vi "flush_debug_fifo_all.vi"(8 "error in (no error)":errorcluster, 11 "Refnum in":T1) -> (0 "error out":errorcluster, 3 "Refnum out":T1)   [LabVIEW 2020]
uses:
  <vilib>/rvi/interface/nirviMethod/nirviMethod.xnode
  <vilib>/FPGAPlugInAG/Dynamic/niLvFpga_ReadFifo_Dynamic.vi
  <vilib>/rvi/errors/niLvFpgaMergeErrorWithErrorCode.vi
  RIG-SPECIFIC FILES/FPGA Refs/FPGA Ref.ctl
panel:
  out "Data 4":u32[](array[numeric])
  out "Elements Remaining 4":u32
  out "Elements Remaining 3":u32
  out "Data 3":u64[](array[numeric])
  out "Data 2":u8[](array[numeric])
  out "Elements Remaining 2":u32
  out "Data":u64[](array[numeric])
  out "Elements Remaining":u32
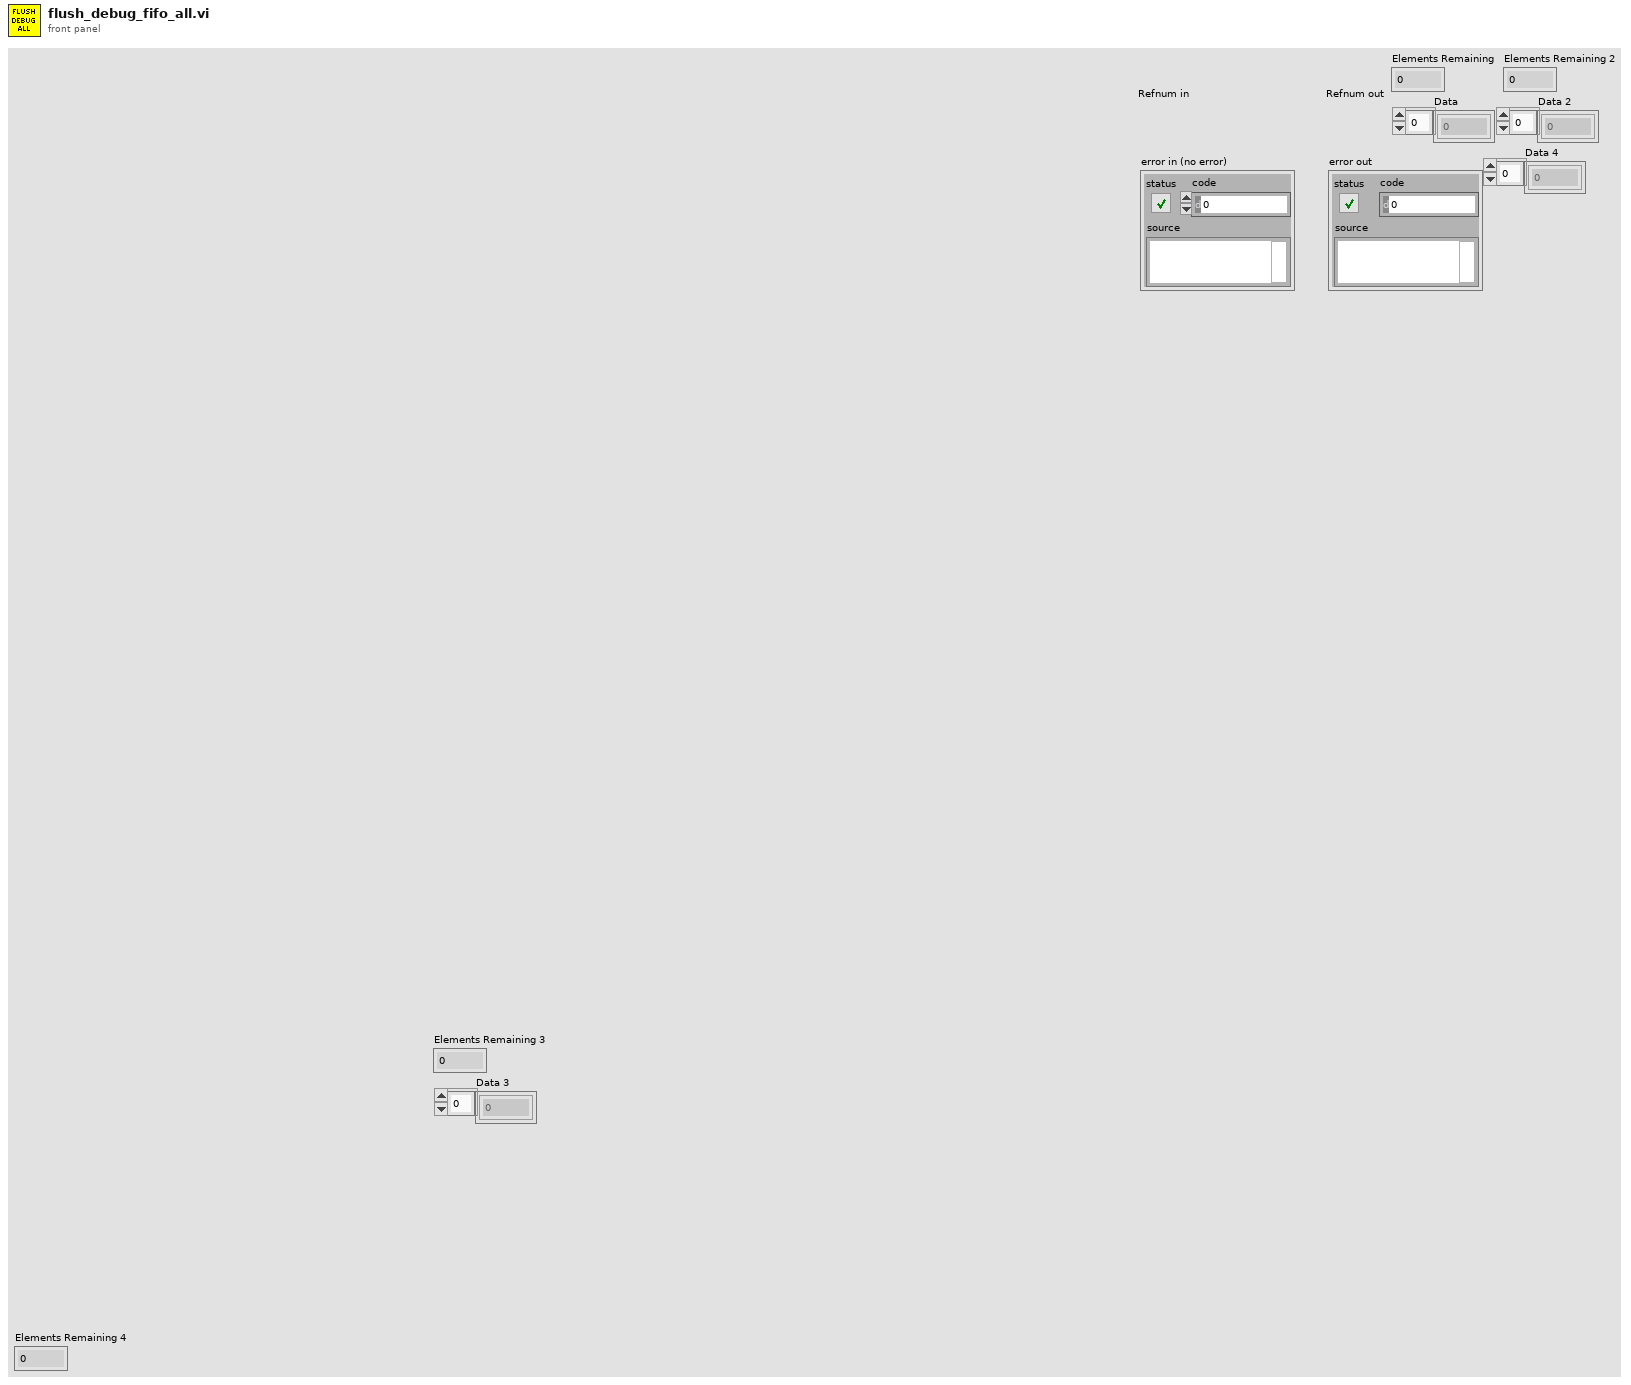
[diagram p1: front panel]
types:
  T1 = typedef "FPGA Ref.ctl" = refnum<k20>
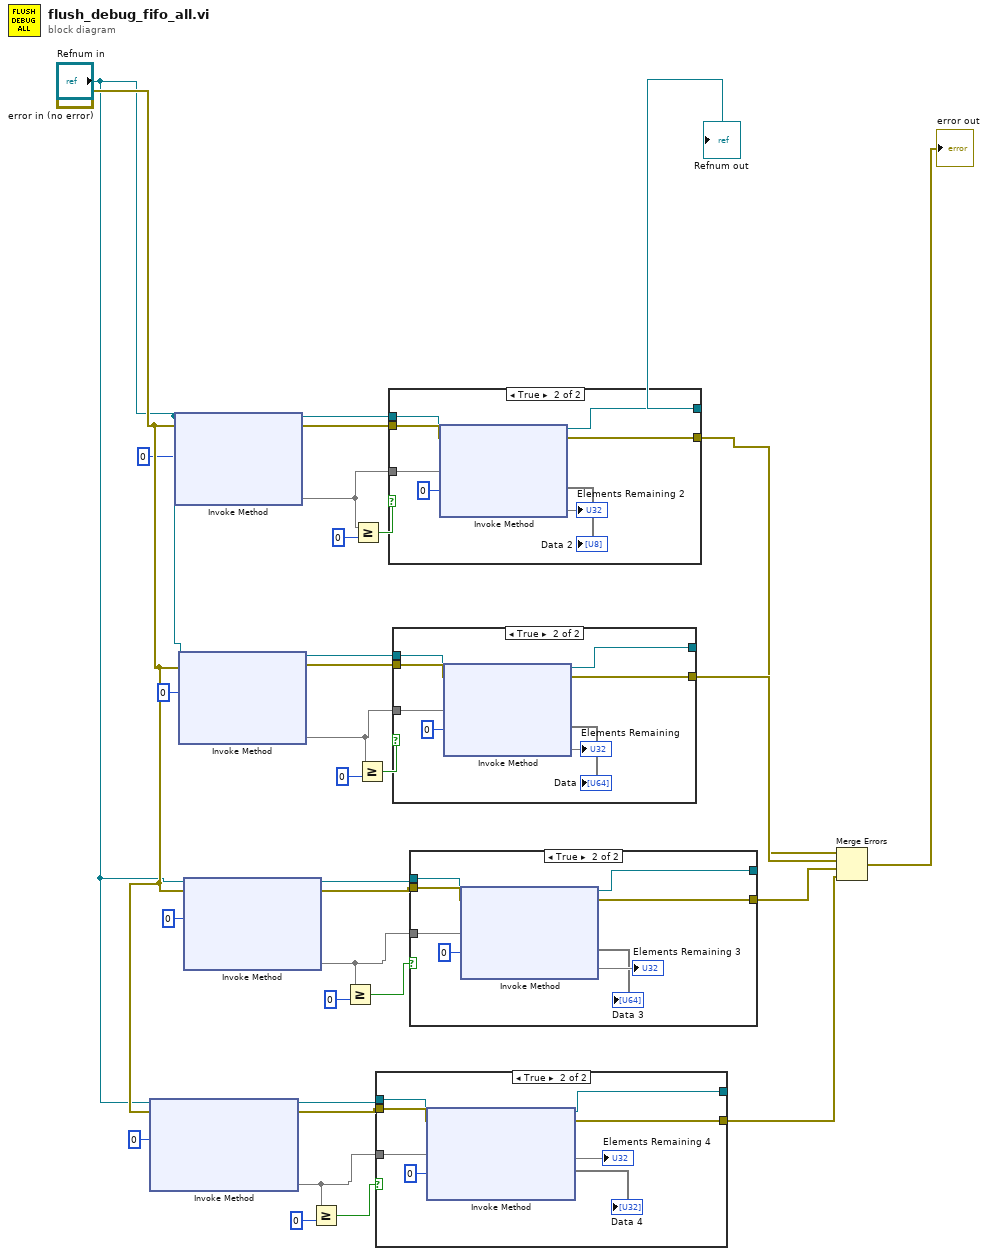
[diagram p0: block diagram]
diagram:
  n1 = xnode "Invoke Method"("FPGA VI Reference In"="Refnum in", "error in"="error in (no error)", "Number of Elements"=u32 0) -> ("FPGA VI Reference Out"=w18:T1, "error out"=w17:errorcluster, "Elements Remaining"=w16)  [unwired: 1 in, 1 out]
  n2 = xnode "Invoke Method"("FPGA VI Reference In"="Refnum in", "error in"="error in (no error)", "Number of Elements"=u32 0) -> ("FPGA VI Reference Out"=w12:T1, "error out"=w11:errorcluster, "Elements Remaining"=w10)  [unwired: 1 in, 1 out]
  n3 = xnode "Invoke Method"("FPGA VI Reference In"="Refnum in", "error in"="error in (no error)", "Number of Elements"=u32 0) -> ("FPGA VI Reference Out"=w6:T1, "error out"=w5:errorcluster, "Elements Remaining"=w3)  [unwired: 1 in, 1 out]
  n4 = xnode "Invoke Method"("FPGA VI Reference In"="Refnum in", "error in"="error in (no error)", "Number of Elements"=u32 0) -> ("FPGA VI Reference Out"=w25:T1, "error out"=w24:errorcluster, "Elements Remaining"=w23)  [unwired: 1 in, 1 out]
  n5 = Greater Or Equal?(x=w16, y=u32 0) -> (x >= y?=w20:bool)
  n6 = Greater Or Equal?(x=w23, y=u32 0) -> (x >= y?=w27:bool)
  n7 = Greater Or Equal?(x=w10, y=u32 0) -> (x >= y?=w9:bool)
  n8 = Greater Or Equal?(x=w3, y=u32 0) -> (x >= y?=w4:bool)
  n9 = case shown="True" w20 {
    tunnel: w16 -> [_ w42]
    tunnel: w17 -> [w33 w40]
    tunnel: w18 -> [w34 w39]
    tunnel: [w34 w38] -> _
    tunnel: [w33 w37] -> w13
    frame False {
    }
    frame True {
      n10 = xnode "Invoke Method"("FPGA VI Reference In"=w39, "error in"=w40, "Number of Elements"=w42, "Timeout (ms)"=0) -> ("FPGA VI Reference Out"=w38:T1, "error out"=w37:errorcluster, "Data"=→"Data 4":void[], "Elements Remaining"=→"Elements Remaining 4")
    }
  }
  n11 = case shown="True" w9 {
    tunnel: w10 -> [_ w52]
    tunnel: w11 -> [w43 w50]
    tunnel: w12 -> [w44 w49]
    tunnel: [w44 w48] -> w32
    tunnel: [w43 w47] -> w29
    frame False {
    }
    frame True {
      n12 = xnode "Invoke Method"("FPGA VI Reference In"=w49, "error in"=w50, "Number of Elements"=w52, "Timeout (ms)"=0) -> ("FPGA VI Reference Out"=w48:T1, "error out"=w47:errorcluster, "Data"=→"Data 2":void[], "Elements Remaining"=→"Elements Remaining 2")
    }
  }
  "Refnum out" <- w32
  n13 = case shown="True" w4 {
    tunnel: w3 -> [_ w62]
    tunnel: w5 -> [w53 w60]
    tunnel: w6 -> [w54 w59]
    tunnel: [w54 w58] -> _
    tunnel: [w53 w57] -> w31
    frame False {
    }
    frame True {
      n14 = xnode "Invoke Method"("FPGA VI Reference In"=w59, "error in"=w60, "Number of Elements"=w62, "Timeout (ms)"=0) -> ("FPGA VI Reference Out"=w58:T1, "error out"=w57:errorcluster, "Data"=→"Data":void[], "Elements Remaining"=→"Elements Remaining")
    }
  }
  n15 = case shown="True" w27 {
    tunnel: w23 -> [_ w72]
    tunnel: w24 -> [w63 w70]
    tunnel: w25 -> [w64 w69]
    tunnel: [w64 w68] -> _
    tunnel: [w63 w67] -> w22
    frame False {
    }
    frame True {
      n16 = xnode "Invoke Method"("FPGA VI Reference In"=w69, "error in"=w70, "Number of Elements"=w72, "Timeout (ms)"=0) -> ("FPGA VI Reference Out"=w68:T1, "error out"=w67:errorcluster, "Data"=→"Data 3":void[], "Elements Remaining"=→"Elements Remaining 3")
    }
  }
  n17 = Merge Errors(w29, w31, w22, w13) -> (→"error out":errorcluster)
